vi "PRF_event_down.vi"(2 "Num_Down":i32, 3 "error in (no error)":errorcluster, 4 "Timeout (ms)":i32, 5 "connection ID out":refnum<k5>) -> (0 "error out":errorcluster, 1 "connection ID out 2":refnum<k5>)   [LabVIEW 2016]
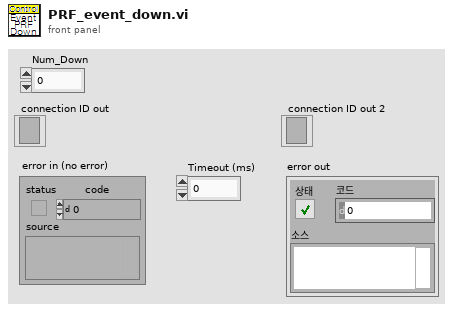
[diagram p1: front panel]
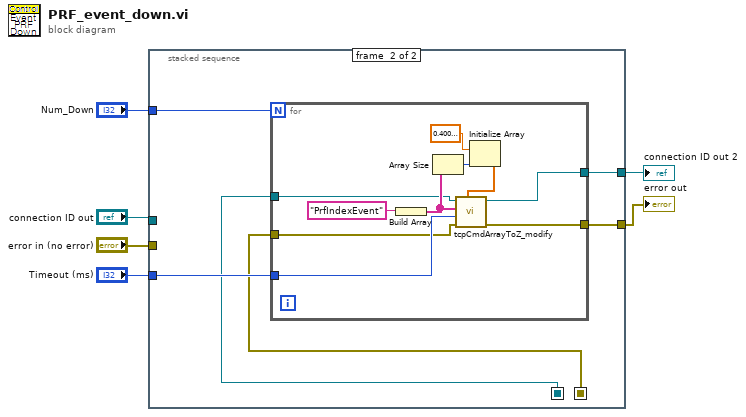
[diagram p0: block diagram]
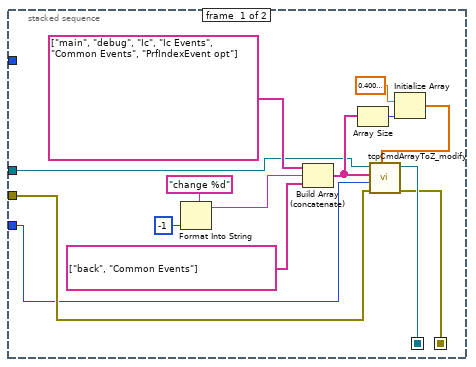
[diagram p2: hidden frame]
diagram:
  n1 = stacked-sequence {
    seq-local: [w8 _] -> [_ w24]
    seq-local: [w7 _] -> [_ w23]
    tunnel: "connection ID out" -> [w11 _]
    tunnel: "error in (no error)" -> [w10 _]
    tunnel: "Timeout (ms)" -> [w9 w26]
    tunnel: [_ w25] -> w6
    tunnel: [_ w22] -> w5
    tunnel: "Num_Down" -> [_ w21]
    frame #0 {
      n2 = Format Into String(format string="change %d" ("Format String"), -1 ("입력 1")) -> (resulting string=w19:string)  [unwired: 2 in, 1 out]
      n3 = Build Array (concatenate)(string[] ["main", "debug", "Ic", "Ic Events", "Common Events", "PrfIndexEvent opt"] ("ROI Minimum"), w19, string[] ["back", "Common Events"] ("ROI")) -> (w16:string[])
      n4 = Array Size(array=w16) -> (size(s)=w12:i32)
      n5 = Initialize Array(sgl 0.4 ("element"), w12) -> (w14:sgl[])
      n6 = call "tcpCmdArrayToZ_modify.vi"("Delay (sec)"=w14, "error in (no error)"=w10, "Timeout (ms)"=w9, "Command array"=w16, "connection ID in"=w11) -> ("error out"=w7:errorcluster, "connection ID out"=w8:refnum<k5>)  [unwired: 2 in, 3 out]
    }
    frame #1 {
      n7 = for {
        N: w21 -> [_]
        tunnel: w24 -> [w32]
        tunnel: w26 -> [w31]
        tunnel: w23 -> [w30]
        tunnel: [w29] -> w25
        tunnel: [w27] -> w22
        n8 = Build Array("PrfIndexEvent") -> (w33:string[])
        n9 = Array Size(array=w33) -> (size(s)=w36:i32)
        n10 = Initialize Array(sgl 0.4 ("element"), w36) -> (w28:sgl[])
        n11 = call "tcpCmdArrayToZ_modify.vi"("Delay (sec)"=w28, "error in (no error)"=w30, "Timeout (ms)"=w31, "Command array"=w33, "connection ID in"=w32) -> ("error out"=w27:errorcluster, "connection ID out"=w29:refnum<k5>)  [unwired: 2 in, 3 out]
      }
    }
  }
  "connection ID out 2" <- w6
  "error out" <- w5
